vi "Get HPS Fault Code Description.vi"(11 "fault code":u64 format="%.0x") -> (3 "fault description":string)   [LabVIEW 2023, in "HPS-17000-PowerModule.lvlib" / "HPS-17000-PowerModule.lvclass"]
uses:
  HPS-17000-PowerModule.lvclass
  ERROR_GLOBAL.ctl
  <vilib>/Utility/error.llb/Trim Whitespace One-Sided.vi
panel:
  in  "FPGA Fault":T1 items=["ERROR_GLOB_EMO_GLOBAL"=0, "ERROR_GLOB_EMO_BUTTON_PRESSED"=1, "ERROR_GLOB_USER"=2, "ERROR_GLOB_PM"=3, "ERROR_GLOB_GRID"=4, "ERROR_GLOB_VOLTAGE_DCBUS_OUT_OF_BOUNDS"=6, "ERROR_GLOB_VOLTAGE_OUTPUT_HIGH"=7, "ERROR_GLOB_VOLTAGE_OUTPUT_LOW"=8, "ERROR_GLOB_VOLTAGE_OUTPUT_UNBALANCE"=9, "ERROR_GLOB_CURRENT_OUTPUT_HIGH"=10, "ERROR_GLOB_SYS_OVERTEMPERATURE"=13, "ERROR_GLOB_SYS_HW"=14, "ERROR_GLOB_SYS_COMM"=15, "ERROR_GLOB_SYNC_AND_CONNECT"=16, "ERROR_GLOB_SP"=20, "ERROR_GLOB_SP_TRACKING"=21, "ERROR_GLOB_CONFIG"=23, "ERROR_GLOB_REG_SYS"=27, "ERROR_GLOB_REG_GRID"=28, "ERROR_GLOB_REG_AFE1"=29, "ERROR_GLOB_REG_AFE2"=30, "ERROR_GLOB_REG_DC"=31]
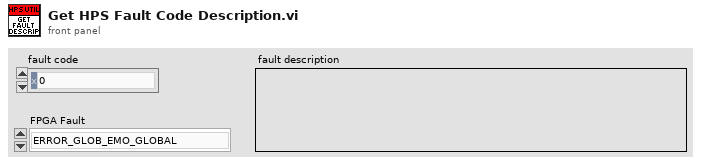
[diagram p1: front panel]
types:
  T1 = typedef "HPS-17000-PowerModule.lvlib/HPS-17000-PowerModule.lvclass/ERROR_GLOBAL.ctl" = u32
  T2 = typedef "LVStringsAndValuesArrayTypeDef_U32.ctl" = cluster{"String":string, "Value":u32}[]
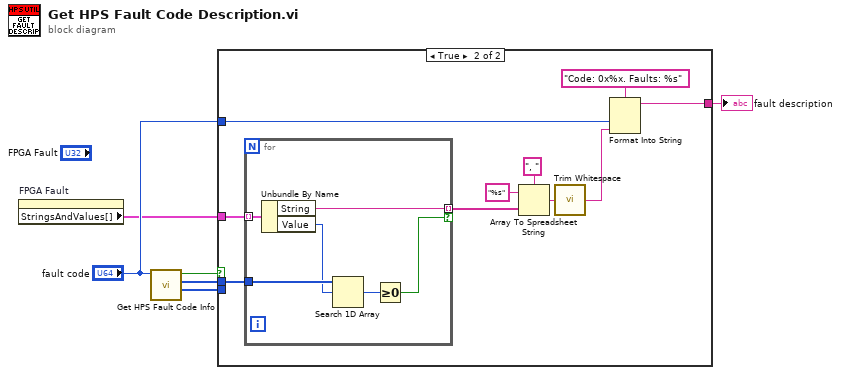
[diagram p0: block diagram]
diagram:
  n1 = property on="FPGA Fault" class="Ring (strict)"() -> ("StringsAndValues[]"=w1:T2)  [unwired: 2 in, 2 out]
  n2 = call "Get HPS Fault Code Info.vi"("fault code"="fault code") -> ("CLIP error bits"=w2:i32[], "fault enums"=w3:T1[], "is fault?"=w4:bool)  [unwired: 8 in]
  n3 = case shown="True" w4 {
    tunnel: w3 -> [_ w16]
    tunnel: w2 -> [_ _]
    tunnel: "fault code" -> [_ w13]
    tunnel: [_ w8] -> w6
    tunnel: w1 -> [_ w7]
    frame False {
    }
    frame True {
      n4 = for {
        tunnel: w16 -> [w21]
        tunnel: [w17] -> w14 mode=indexing if=w22
        tunnel: w7 -> [w20] mode=indexing
        n5 = Unbundle By Name(w20) -> ("String"=w17:string, "Value"=w19:u32)
        n6 = Search 1D Array(1D array=w21, element=w19) -> (index of element=w18:i32)  [unwired: 1 in]
        n7 = Greater Or Equal To 0?(x=w18) -> (x >= 0?=w22:bool)
      }
      n8 = Array To Spreadsheet String(delimiter (Tab)=", ", array=w14, 3:"%s" ("format string")) -> (spreadsheet string=w10:string)
      n9 = call <vilib>:"Trim Whitespace.vi"("string"=w10) -> ("trimmed string"=w9:string)  [unwired: 1 in]
      n10 = Format Into String(format string="Code: 0x%x. Faults: %s", w13, w9) -> (resulting string=w8:string)  [unwired: 2 in, 1 out]
    }
  }
  "fault description" <- w6
